vi "CANShark_DeviceOpen.vi"(9 "error in (no error)":errorcluster, 10 "Device Index":i32, 11 "Mode":i32) -> (2 "error out":errorcluster, 3 "CANSHARK_DEVICE":i64)   [LabVIEW 2026]
uses:
  x64/Release/CanSharkApi_Dll1.dll
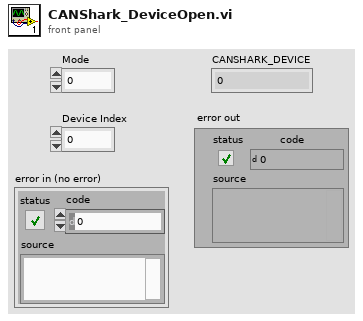
[diagram p1: front panel]
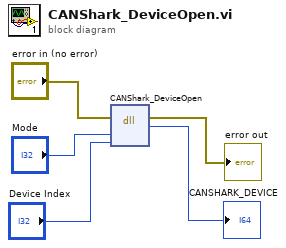
[diagram p0: block diagram]
diagram:
  n1 = dll-call lib="C:/Users/TECQNIO/Documents/CANSHARK LABVIEW API PACKAGE/x64/Release/CanSharkApi_Dll1.dll" fn="CANShark_DeviceOpen"(error in="error in (no error)", "Mode"="Mode", "deviceIndex"="Device Index") -> (error out=→"error out":errorcluster, "return type"=→"CANSHARK_DEVICE":i64)  [unwired: 4 in, 1 out]
